vi "AddAlarmMeasurement.vi"(6 "OID Numbers":string[](array[string]), 7 "Model Information":string[][](array[string]), 8 "Error In":errorcluster, 11 "Measurements To Read Array In":u16[](array[numeric])) -> (0 "Error Out":errorcluster, 3 "Measurements To Read Array Out":u16[](array[numeric]))   [LabVIEW 2018, in "SensorPlugins.lvlib" / "RoomAlert.lvclass"]
doc: "Adds an alarm measurement to ensure the RoomAlert plugin is always checking if an alarm occured."
uses:
  RoomAlert.lvclass
  <vilib>/Utility/error.llb/Error Cluster From Error Code.vi
  <vilib>/ErrorRing/Error Ring.xnode
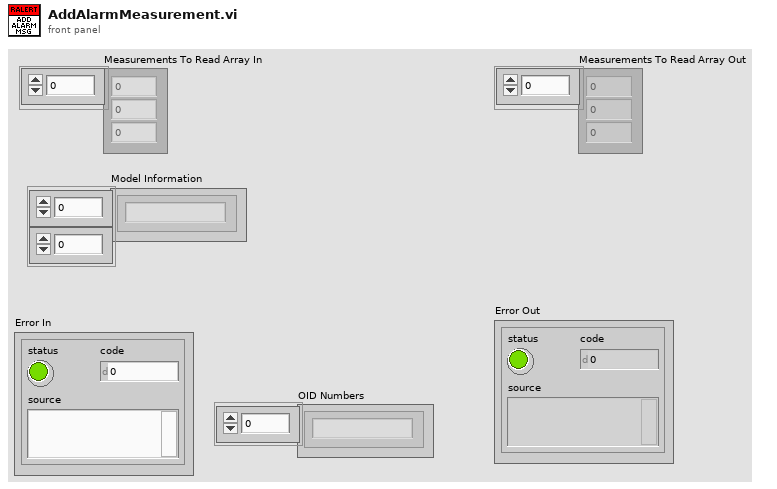
[diagram p1: front panel]
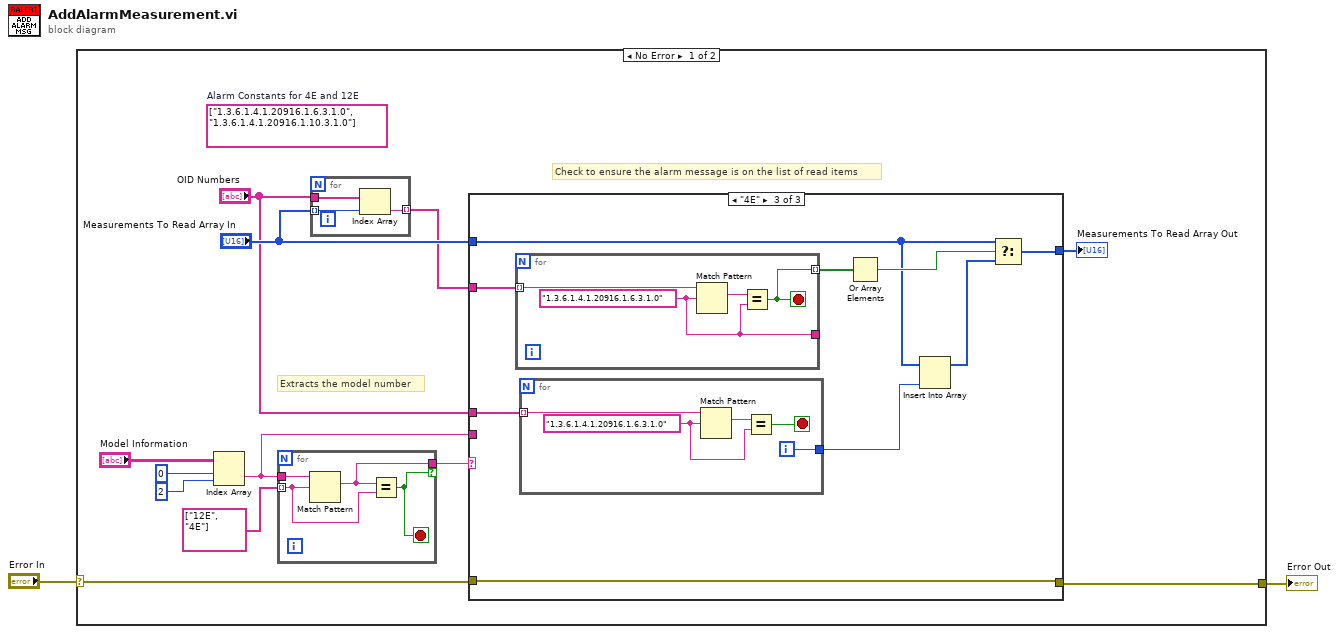
[diagram p0: block diagram]
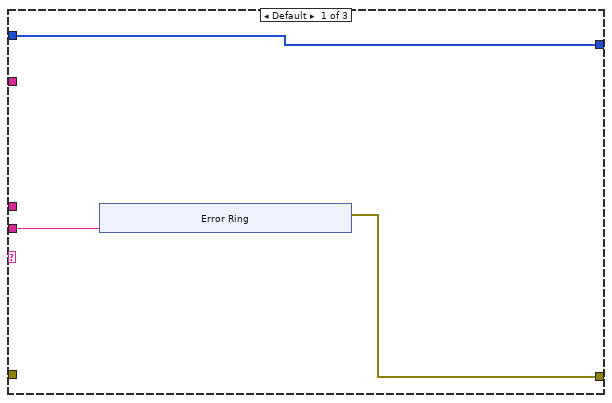
[diagram p2: hidden frame]
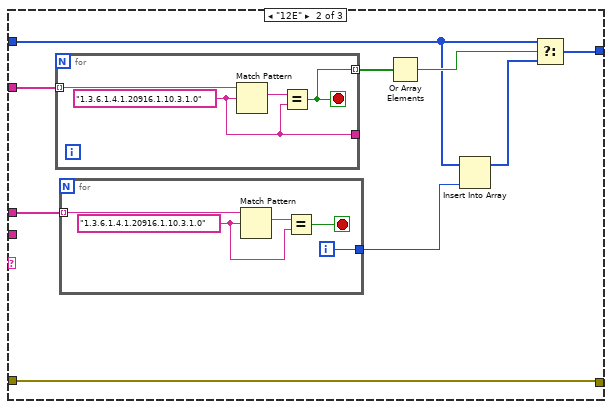
[diagram p3: hidden frame]
diagram:
  n1 = case shown="No Error" "Error In" {
    selector: "Error In" -> [w10 w68]
    tunnel: [w9 w68] -> w1
    frame No Error {
      (unwired) string[] ["1.3.6.1.4.1.20916.1.6.3.1.0", "1.3.6.1.4.1.20916.1.10.3.1.0"]  # Alarm Constants for 4E and 12E
      # "Extracts the model number"
      # "Check to ensure the alarm message is on the list of read items"
      n2 = Index Array(array="Model Information", index (row)=0, index (col)=2 ("disabled index (col)")) -> (element=w3:string)
      n3 = for {
        tunnel: w3 -> [w18]
        tunnel: string[] ["12E", "4E"] -> [w17] mode=indexing
        tunnel: [w16] -> w4 if=w15
        stop <- w15 stop-if-true
        n4 = Match Pattern(string=w18, regular expression=w17) -> (match substring=w16:string)  [unwired: 1 in, 3 out]
        n5 = Equal?(x=w16, y=w17) -> (x = y?=w15:bool)
      }
      n6 = for {
        tunnel: "Measurements To Read Array In" -> [w20] mode=indexing
        tunnel: "OID Numbers" -> [w21]
        tunnel: [w19] -> w7 mode=indexing
        n7 = Index Array(array=w21, index=w20) -> (element=w19:string)
      }
      n8 = case shown="\"4E\"" w4 {
        tunnel: "Measurements To Read Array In" -> [w24 w34 w52]
        tunnel: [w24 w36 w54] -> w14
        tunnel: w10 -> [_ w40 w58]
        tunnel: [w23 w40 w58] -> w9
        tunnel: w7 -> [_ w39 w57]
        tunnel: "OID Numbers" -> [_ w35 w53]
        tunnel: w3 -> [w22 _ _]
        frame Default {
          n9 = xnode "Error Ring"("parameter 0"=w22) -> ("error out"=w23:errorcluster)
        }
        frame "12E" {
          n10 = for {
            tunnel: w39 -> [w49] mode=indexing
            tunnel: [w47] -> w38 mode=indexing
            tunnel: [w46] -> _
            stop <- w47 stop-if-true
            w46 = "1.3.6.1.4.1.20916.1.10.3.1.0" ("regular expression")
            n11 = Match Pattern(string=w49, regular expression=w46) -> (match substring=w48:string)  [unwired: 1 in, 3 out]
            n12 = Equal?(x=w48, y=w46) -> (x = y?=w47:bool)
          }
          n13 = for {
            tunnel: w35 -> [w45] mode=indexing
            tunnel: [w41] -> w33
            i -> [w41]
            stop <- w43 stop-if-true
            w42 = "1.3.6.1.4.1.20916.1.10.3.1.0" ("regular expression")
            n14 = Match Pattern(string=w45, regular expression=w42) -> (match substring=w44:string)  [unwired: 1 in, 3 out]
            n15 = Equal?(x=w44, y=w42) -> (x = y?=w43:bool)
          }
          n16 = Or Array Elements(Boolean array=w38) -> (logical OR=w37:bool)
          n17 = Insert Into Array(array=w34, new element=w33) -> (w32:u16[])  [unwired: 1 in]
          n18 = Select(t=w34, s=w37, f=w32) -> (s? t:f=w36:u16[])
        }
        frame "4E" {
          n19 = for {
            tunnel: w57 -> [w67] mode=indexing
            tunnel: [w65] -> w56 mode=indexing
            tunnel: [w64] -> _
            stop <- w65 stop-if-true
            w64 = "1.3.6.1.4.1.20916.1.6.3.1.0" ("regular expression")
            n20 = Match Pattern(string=w67, regular expression=w64) -> (match substring=w66:string)  [unwired: 1 in, 3 out]
            n21 = Equal?(x=w66, y=w64) -> (x = y?=w65:bool)
          }
          n22 = for {
            tunnel: w53 -> [w63] mode=indexing
            tunnel: [w59] -> w51
            i -> [w59]
            stop <- w61 stop-if-true
            w60 = "1.3.6.1.4.1.20916.1.6.3.1.0" ("regular expression")
            n23 = Match Pattern(string=w63, regular expression=w60) -> (match substring=w62:string)  [unwired: 1 in, 3 out]
            n24 = Equal?(x=w62, y=w60) -> (x = y?=w61:bool)
          }
          n25 = Or Array Elements(Boolean array=w56) -> (logical OR=w55:bool)
          n26 = Insert Into Array(array=w52, new element=w51) -> (w50:u16[])  [unwired: 1 in]
          n27 = Select(t=w52, s=w55, f=w50) -> (s? t:f=w54:u16[])
        }
      }
      "Measurements To Read Array Out" <- w14
    }
    frame Error {
    }
  }
  "Error Out" <- w1
